vi "Format Indent.vi"(9 "Indent":i32, 11 "IPersist in":refnum<class "IPersist.lvclass">) -> (1 "Indent out":i32, 3 "IPersist out":refnum<class "IPersist.lvclass">, 4 "Indent XML":string)   [LabVIEW 2020, in "IPersist.lvlib" / "IPersist.lvclass"]
uses:
  <vilib>/gpm_packages/@cs/persistence/source/IPersist/IPersist.lvclass
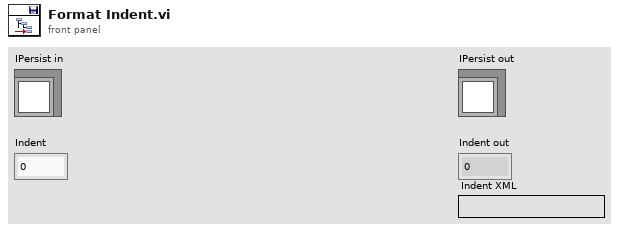
[diagram p1: front panel]
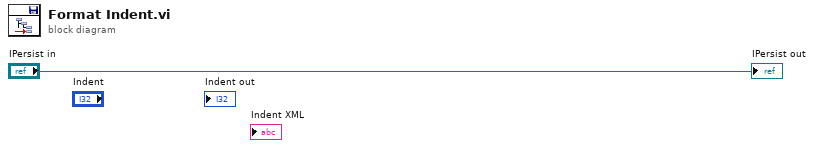
[diagram p0: block diagram]
diagram:
  "IPersist out" <- "IPersist in"
